vi "Cylinder_Finished.vi"(3 "Value_Changed?":bool) -> (1 "Finished?":bool)   [LabVIEW 2016]
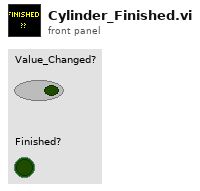
[diagram p1: front panel]
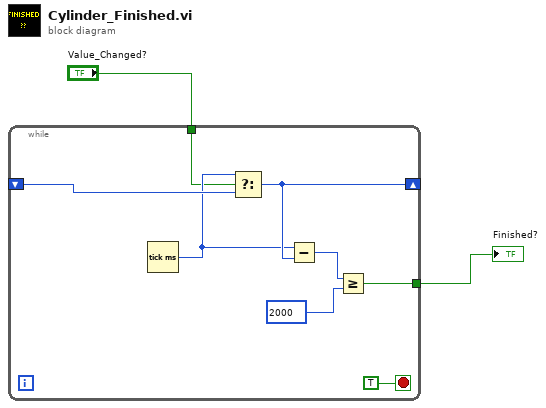
[diagram p0: block diagram]
diagram:
  n1 = while {
    shift-right: [w5] -> _
    shift-left: _ -> [w6]
    tunnel: [w8] -> w2
    tunnel: "Value_Changed?" -> [w3]
    stop <- TRUE stop-if-true
    n2 = Tick Count (ms)() -> (millisecond timer value=w4:u32)
    n3 = Select(t=w4, s=w3, f=w6) -> (s? t:f=w5:u32)
    n4 = Subtract(x=w4, y=w5) -> (x-y=w9:u32)
    n5 = Greater Or Equal?(x=w9, y=u32 2000) -> (x >= y?=w8:bool)
  }
  "Finished?" <- w2
